vi "3.7-Establish UDP.vi"() -> ()   [LabVIEW 2010]
uses:
  4-High Neurons/4.1-Act Control Typedef.ctl
  4-High Neurons/4.1.0-Datatype Typedef.ctl
  3.0-Global.vi
panel:
  out "error out":errorcluster
  out "String 2":string
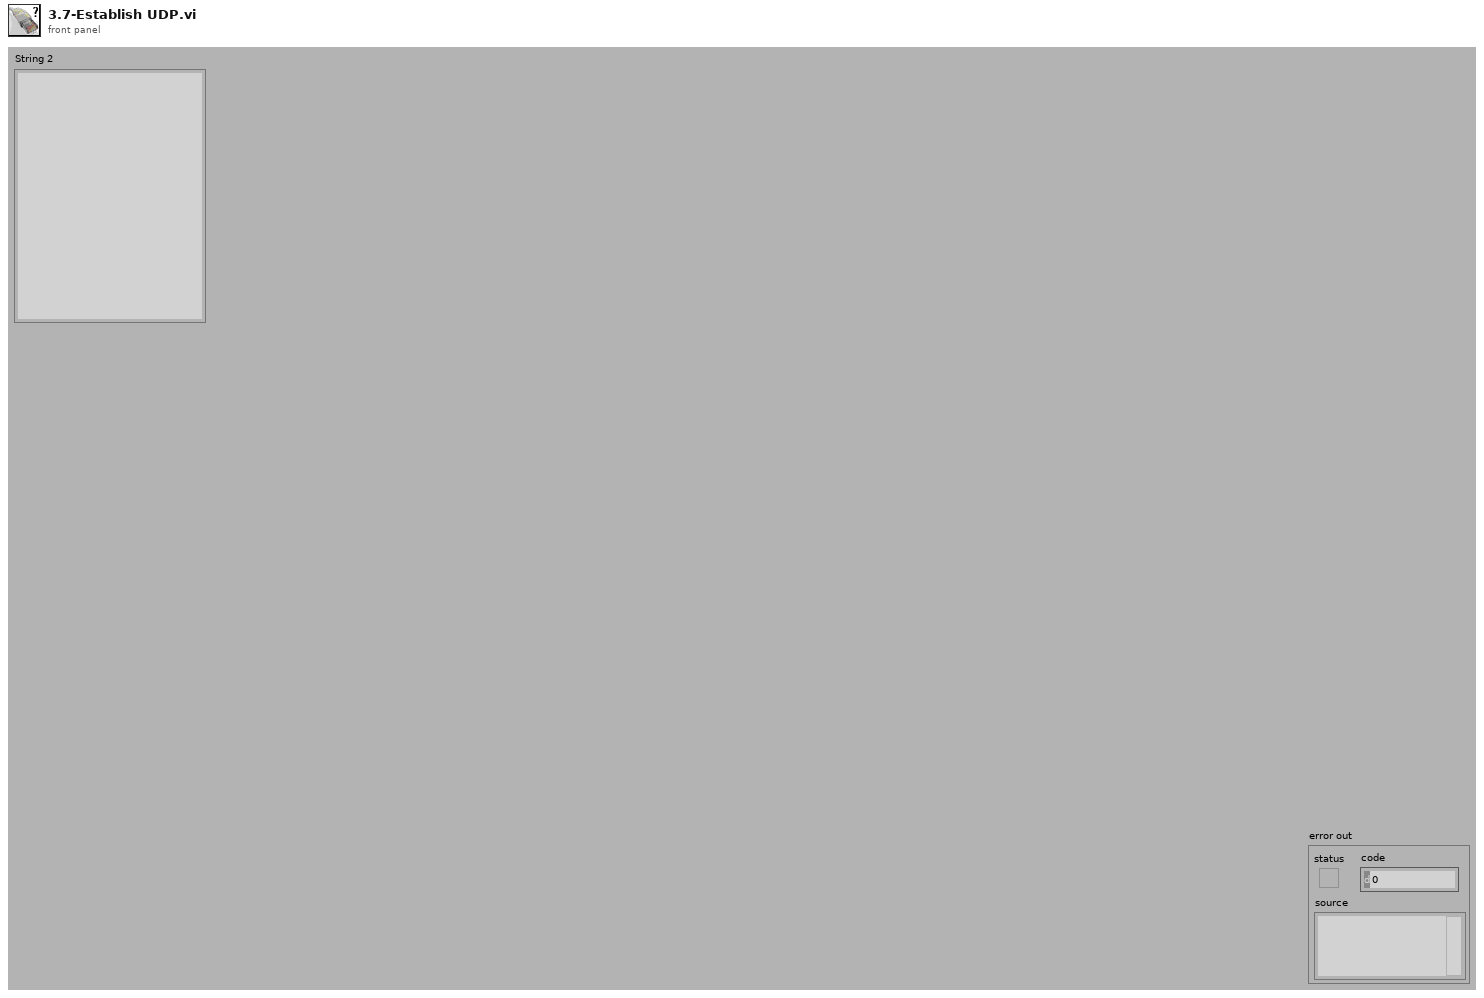
[diagram p1: front panel]
types:
  T1 = typedef "4.1-Act Control Typedef.ctl" = cluster{"4.1.0 Data":variant, "Type of Data":T2, "E-Stop":bool, "Restart":bool, "New IP":bool, "Begin":bool, "Time":i32, "Shutdown":bool}
  T2 = typedef "4.1.0-Datatype Typedef.ctl" = enum16{"4.1.0-Empty Data", "4.1.1-Joystick Data", "4.1.2-Behavioral Data"}
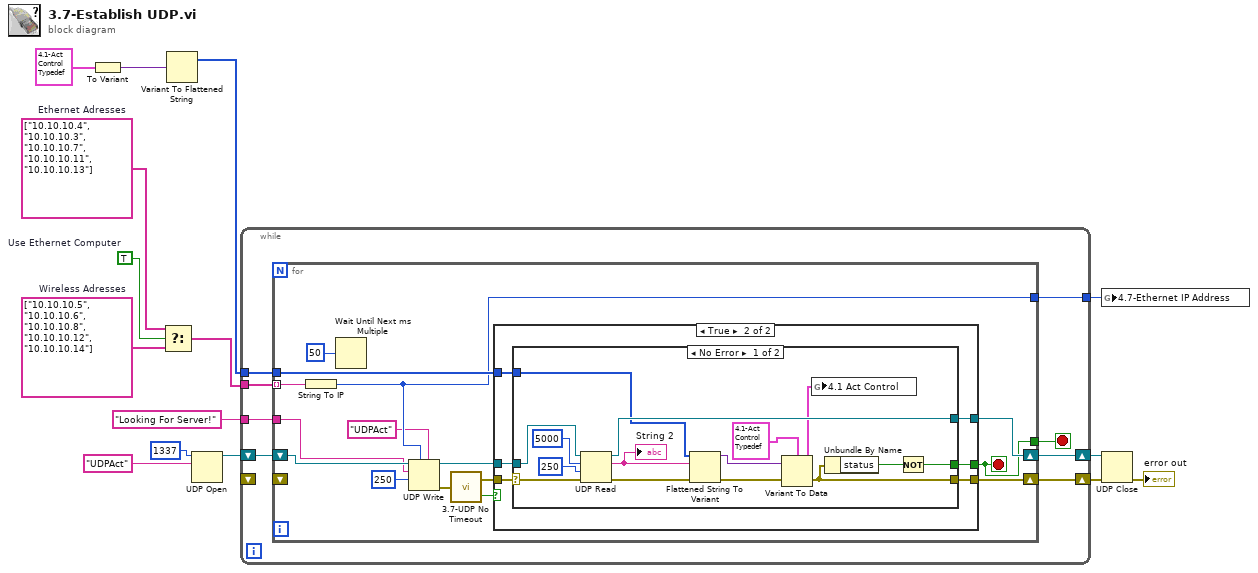
[diagram p0: block diagram]
diagram:
  w11 = TRUE  # Use Ethernet Computer
  w12 = string[] ["10.10.10.5", "10.10.10.6", "10.10.10.8", "10.10.10.12", "10.10.10.14"]  # Wireless Adresses
  w13 = string[] ["10.10.10.4", "10.10.10.3", "10.10.10.7", "10.10.10.11", "10.10.10.13"]  # Ethernet Adresses
  n1 = To Variant(anything=T1 {"4.1.0 Data"=variant, "Type of Data"=enum."4.1.0-Empty Data", "E-Stop"=FALSE, "Restart"=FALSE, "New IP"=FALSE, "Begin"=FALSE, "Time"=0, "Shutdown"=FALSE} ("4.1 Act Control")) -> (Variant=w15:variant)
  n2 = Select(t=w13, s=w11, f=w12) -> (s? t:f=w10:string[])
  n3 = Variant To Flattened String(Variant=w15) -> (1:w7:i16[])  [unwired: 1 out]
  n4 = UDP Open(10:"UDPAct", 11:u16 1337 ("port")) -> (port=w8:refnum<k16>)  [unwired: 3 in, 2 out]
  n5 = while {
    tunnel: w10 -> [w23]
    shift-right: [w20] -> w5
    shift-left: w8 -> [w21]
    tunnel: w7 -> [w19]
    shift-right: [w18] -> w4
    shift-left: _ -> [_]
    tunnel: "Looking For Server!" -> [w17]
    tunnel: [w16] -> w1
    stop <- w22 stop-if-true
    n6 = for {
      tunnel: w23 -> [w38] mode=indexing
      tunnel: [w27] -> w22
      shift-right: [w32] -> w20
      shift-left: w21 -> [w37]
      tunnel: w19 -> [w29]
      shift-right: [w28] -> w18
      shift-left: _ -> [_]
      tunnel: w17 -> [w26]
      tunnel: [w25] -> w16
      stop <- w27 stop-if-true
      n7 = String To IP(1:w38) -> (0:w25:u32)
      n8 = Wait Until Next ms Multiple(millisecond multiple=u32 50) -> ()  [unwired: 1 out]
      n9 = UDP Write(address=w25, port or service name="UDPAct", connection ID=w37, data in=w26, 9:250 ("timeout ms (25000)")) -> (error out=w35:errorcluster, 3:w33:refnum<k16>)  [unwired: 1 in]
      n10 = call "3.7-UDP No Timeout.vi"("error in (no error)"=w35) -> ("No Timeout"=w30:bool, "error out"=w31:errorcluster)
      n11 = case shown="True" w30 {
        tunnel: w31 -> [w40 w46]
        tunnel: w33 -> [w39 w45]
        tunnel: [w39 w44] -> w32
        tunnel: [w40 w43] -> w28
        tunnel: w29 -> [_ w42]
        tunnel: [_ w41] -> w27
        frame False {
        }
        frame True {
          n12 = case shown="No Error" w46 {
            selector: w46 -> [w61 w62]
            tunnel: w45 -> [w60 w63]
            tunnel: [w58 w63] -> w44
            tunnel: [w50 w62] -> w43
            tunnel: w42 -> [w55 _]
            tunnel: [w48 _] -> w41
            frame No Error {
              n13 = UDP Read(connection ID=w60, max size (548)=5000, timeout ms (25000)=250, 8:w61) -> (data out=w56:string, error out=w51:errorcluster, 3:w58:refnum<k16>)  [unwired: 2 out]
              "String 2" <- w56
              n14 = Flattened String To Variant(4:w51, 6:w56, 7:w55) -> (0:w52:errorcluster, 3:w54:variant)
              n15 = Variant To Data(error in=w52, Variant=w54, type=T1 {"4.1.0 Data"=variant, "Type of Data"=enum."4.1.1-Joystick Data", "E-Stop"=FALSE, "Restart"=FALSE, "New IP"=FALSE, "Begin"=FALSE, "Time"=0, "Shutdown"=FALSE} ("4.1 Act Control")) -> (error out=w50:errorcluster, data=w47:T1)
              n16 = global write "3.0-Global.vi" "4.1 Act Control"(w47) -> ()
              n17 = Unbundle By Name(w50) -> ("status"=w49:bool)
              n18 = Not(x=w49) -> (.not. x?=w48:bool)
            }
            frame Error {
            }
          }
        }
      }
    }
  }
  n19 = global write "3.0-Global.vi" "4.7-Ethernet IP Address"(w1) -> ()
  n20 = UDP Close(connection ID=w5, 8:w4) -> (error out=→"error out":errorcluster)  [unwired: 1 out]
